vi "Configure ARM Layer.vi"(0 "VISA resource name":refnum<visa-resource-name>, 1 "ARM Timer Interval (2E-5 seconds)":dbl=2e-05, 2 "ARM Source (0: Auto-Internal)":i32(ring) items=["Auto-Internal", "BUS", "Timer", "INT1", "INT2", "LAN", "EXT1", "EXT2", "EXT3", "EXT4", "EXT5", "EXT6", "EXT7", "EXT8", "EXT9", "EXT10", "EXT11", "EXT12", "EXT13", "EXT14"], 3 "Device Action (2: Both)":i32(ring)=2 items=["Acquire", "Transient", "Both"], 5 "Channel (0: Channel 1)":i32(ring) items=["Channel 1", "Channel 2"], 7 "ARM Delay (0 second)":dbl, 9 "ARM Count (1)":dbl=1.0, 11 "error in (no error)":errorcluster, 12 "ARM Bypass Mode (1: Off)":i32(ring)=1 items=["Once", "Off"], 13 "LXI Triggers For ARM Trigger":bool[](array[boolean])=[TRUE, TRUE, TRUE, TRUE, TRUE, TRUE, TRUE, TRUE]) -> (4 "VISA resource name out":refnum<visa-resource-name>, 15 "error out":errorcluster)   [LabVIEW 2020, in "Agilent B2900 Series.lvlib"]
doc: "The ARM-Trigger model shows independent event detection for the ARM and Trigger layers. This VI configures ARM layer in ARM-Trigger model."
uses:
  Agilent B2900 Series.lvlib
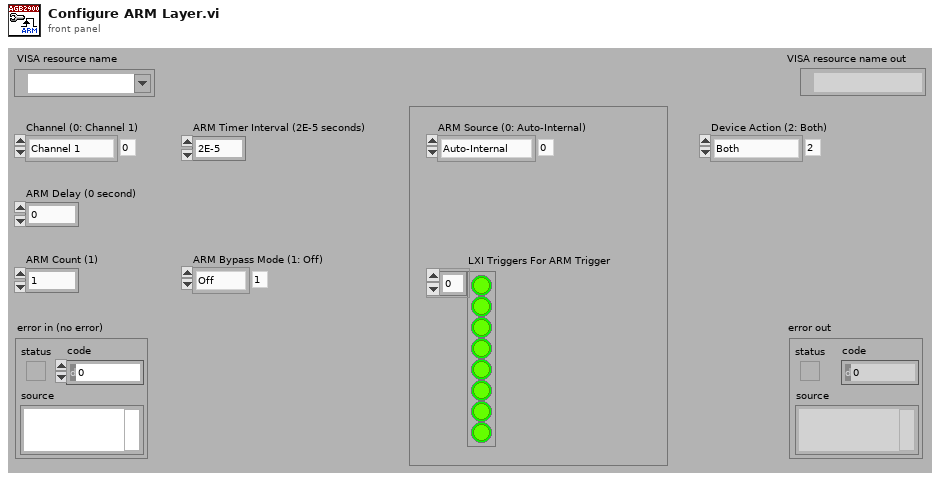
[diagram p1: front panel]
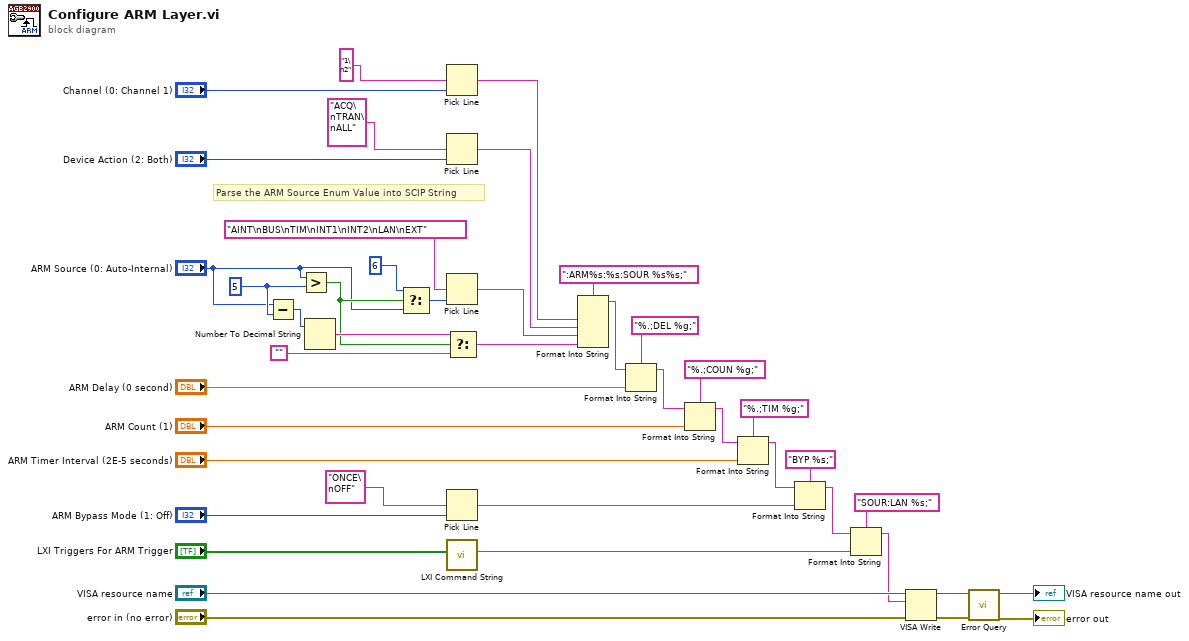
[diagram p0: block diagram]
diagram:
  w22 = 5 ("y")
  # "Parse the ARM Source Enum Value into SCIP String"
  n1 = Subtract(x="ARM Source (0: Auto-Internal)", y=w22) -> (x-y=w7:i32)
  n2 = Greater?(x="ARM Source (0: Auto-Internal)", y=w22) -> (0:w8:bool)
  n3 = Number To Decimal String(number=w7) -> (decimal integer string=w10:string)  [unwired: 1 in]
  n4 = Select(t=6 ("f"), s=w8, f="ARM Source (0: Auto-Internal)") -> (s? t:f=w9:i32)
  n5 = Pick Line(multi-line string="1\n2" ("string (\"\")"), line index="Channel (0: Channel 1)") -> (output string=w24:string)  [unwired: 1 in]
  n6 = Pick Line(multi-line string="ACQ\nTRAN\nALL" ("string (\"\")"), line index="Device Action (2: Both)") -> (output string=w25:string)  [unwired: 1 in]
  n7 = Pick Line(multi-line string="AINT\nBUS\nTIM\nINT1\nINT2\nLAN\nEXT", line index=w9) -> (output string=w23:string)  [unwired: 1 in]
  n8 = Pick Line(multi-line string="ONCE\nOFF", line index="ARM Bypass Mode (1: Off)") -> (output string=w13:string)  [unwired: 1 in]
  n9 = call "LXI Command String.vi"("LXI Triggers"="LXI Triggers For ARM Trigger") -> ("LXI Command String"=w3:string)  [unwired: 10 in]
  n10 = Select(t=w10, s=w8, f="") -> (s? t:f=w20:string)
  n11 = Format Into String(format string=":ARM%s:%s:SOUR %s%s;" ("string (\"\")"), w24, w25, w23, w20) -> (resulting string=w19:string)  [unwired: 2 in, 1 out]
  n12 = Format Into String(format string="%.;DEL %g;", initial string=w19, "ARM Delay (0 second)") -> (resulting string=w18:string)  [unwired: 1 in, 1 out]
  n13 = Format Into String(format string="%.;COUN %g;", initial string=w18, "ARM Count (1)") -> (resulting string=w17:string)  [unwired: 1 in, 1 out]
  n14 = Format Into String(format string="%.;TIM %g;", initial string=w17, "ARM Timer Interval (2E-5 seconds)") -> (resulting string=w14:string)  [unwired: 1 in, 1 out]
  n15 = Format Into String(format string="BYP %s;", initial string=w14, w13) -> (resulting string=w12:string)  [unwired: 1 in, 1 out]
  n16 = Format Into String(format string="SOUR:LAN %s;", initial string=w12, w3) -> (resulting string=w1:string)  [unwired: 1 in, 1 out]
  n17 = VISA Write(VISA resource name="VISA resource name", write buffer=w1, error in (no error)="error in (no error)") -> (VISA resource name out=w35:refnum<visa-resource-name>, error out=w34:errorcluster)  [unwired: 1 out]
  n18 = call "Error Query.vi"("error in (no error)"=w34, "VISA resource name"=w35) -> ("error out"=→"error out":errorcluster, "VISA resource name out"=→"VISA resource name out":refnum<visa-resource-name>)  [unwired: 6 in, 2 out]
